vi "DOE Calculate Dryer EF.vi"(5 "Use Runtime RMC Calculation?":bool=TRUE, 7 "Dryer Initial IMC Data in":T7 {"Maximum Weight (lbf)" format="%03_6g"; "Average Weight (lbf)" format="%03_6g"; "Minimum Weight (lbf)" format="%03_6g"; "CEF (lbf/kWh)" format="%03_6g"; "Actual Final RMC (%)" format="%03_6g"; "Tolerance(%)" format="%0#_6g"; "Bone Dry Wt(lbs)" format="%03_6g"; "RMC (Desired %)" format="%0#_6g"; "Actual Initial RMC (%)" format="%03_6g"; "Measured IMC (lbs)" format="%0#_6g"}, 8 "Error In":errorcluster, 11 "Measurments":T1 {"Power Measurements"."Voltage (V):Element 1 Avg" format="%.3g"; "Power Measurements"."Voltage (V):Element 2 Avg" format="%.3g"; "Power Measurements"."Max Watt Hours" format="%.3g"; "Power Measurements"."Power Factor:Element 2" format="%.3g"; "Power Measurements"."Power Factor:Element 1" format="%.3g"; "Power Measurements"."Apparent Power (VA):Element 2" format="%.3g"; "Power Measurements"."Apparent Power (VA):Element 1" format="%.3g"; "Power Measurements"."Frequency (Hz):Element 1" format="%.3g"; "Power Measurements"."Time:Element 1" format="%.3g"; "Power Measurements"."Voltage Crest Factor:Element 2" format="%.3g"; "Power Measurements"."Voltage Crest Factor:Element 1" format="%.3g"; "Power Measurements"."Voltage Harmonic (%):Element 2" format="%.3g"; "Power Measurements"."Voltage Harmonic (%):Element 1" format="%.3g"; "Power Measurements"."Current Crest Factor:Element 2" format="%.3g"; "Power Measurements"."Current Crest Factor:Element 1" format="%.3g"; "Power Measurements"."Voltage (V):Element 1" format="%.3g"; "Power Measurements"."Voltage (V):Element 2" format="%.3g"; "Power Measurements"."Watt Hours (Wh):Sigma" format="%.3f"; "Power Measurements"."Power (W):Sigma" format="%.3g"; "Power Measurements"."Current (A):Element 2" format="%.3e"; "Power Measurements"."Current (A):Element 1" format="%.3e"}) -> (0 "Error Out":errorcluster, 1 "RMC Data":string[][](array[string]), 2 "Dryer Initial IMC Data out":T7 {"Maximum Weight (lbf)" format="%03_6g"; "Average Weight (lbf)" format="%03_6g"; "Minimum Weight (lbf)" format="%03_6g"; "CEF (lbf/kWh)" format="%03_6g"; "Actual Final RMC (%)" format="%03_6g"; "Tolerance(%)" format="%0#_6g"; "Bone Dry Wt(lbs)" format="%03_6g"; "RMC (Desired %)" format="%0#_6g"; "Actual Initial RMC (%)" format="%03_6g"; "Measured IMC (lbs)" format="%0#_6g"}, 3 "Measurments Out":T1 {"Power Measurements"."Voltage (V):Element 1 Avg" format="%.3g"; "Power Measurements"."Voltage (V):Element 2 Avg" format="%.3g"; "Power Measurements"."Max Watt Hours" format="%.3g"; "Power Measurements"."Power Factor:Element 2" format="%.3g"; "Power Measurements"."Power Factor:Element 1" format="%.3g"; "Power Measurements"."Apparent Power (VA):Element 2" format="%.3g"; "Power Measurements"."Apparent Power (VA):Element 1" format="%.3g"; "Power Measurements"."Frequency (Hz):Element 1" format="%.3g"; "Power Measurements"."Time:Element 1" format="%.3g"; "Power Measurements"."Voltage Crest Factor:Element 2" format="%.3g"; "Power Measurements"."Voltage Crest Factor:Element 1" format="%.3g"; "Power Measurements"."Voltage Harmonic (%):Element 2" format="%.3g"; "Power Measurements"."Voltage Harmonic (%):Element 1" format="%.3g"; "Power Measurements"."Current Crest Factor:Element 2" format="%.3g"; "Power Measurements"."Current Crest Factor:Element 1" format="%.3g"; "Power Measurements"."Voltage (V):Element 1" format="%.3g"; "Power Measurements"."Voltage (V):Element 2" format="%.3g"; "Power Measurements"."Watt Hours (Wh):Sigma" format="%.3f"; "Power Measurements"."Power (W):Sigma" format="%.3g"; "Power Measurements"."Current (A):Element 2" format="%.3e"; "Power Measurements"."Current (A):Element 1" format="%.3e"})   [LabVIEW 2020]
uses:
  Type Definitions/DOE Front Panel Meters.ctl
  Utility/Type Definitions/UTILITY Power Data.ctl
  Utility/Standby Power/Type Definitions/Standby Power Main Data.ctl
  Drivers/Omega FMA-1600A Series Gas Flow Meter/Type Definitions/FMA1600A Gas Data.ctl
  Drivers/Omega FMA-1600A Series Gas Flow Meter/Type Definitions/FMA1600A Gas Type.ctl
  Range/Type Definitions/RANGE Meter Selector 1-2.ctl
  Utility/Save File/File Setup (Public)/Type Definition/DPT IMC Data.ctl
  Type Definitions/DOE Dryer Standard.ctl
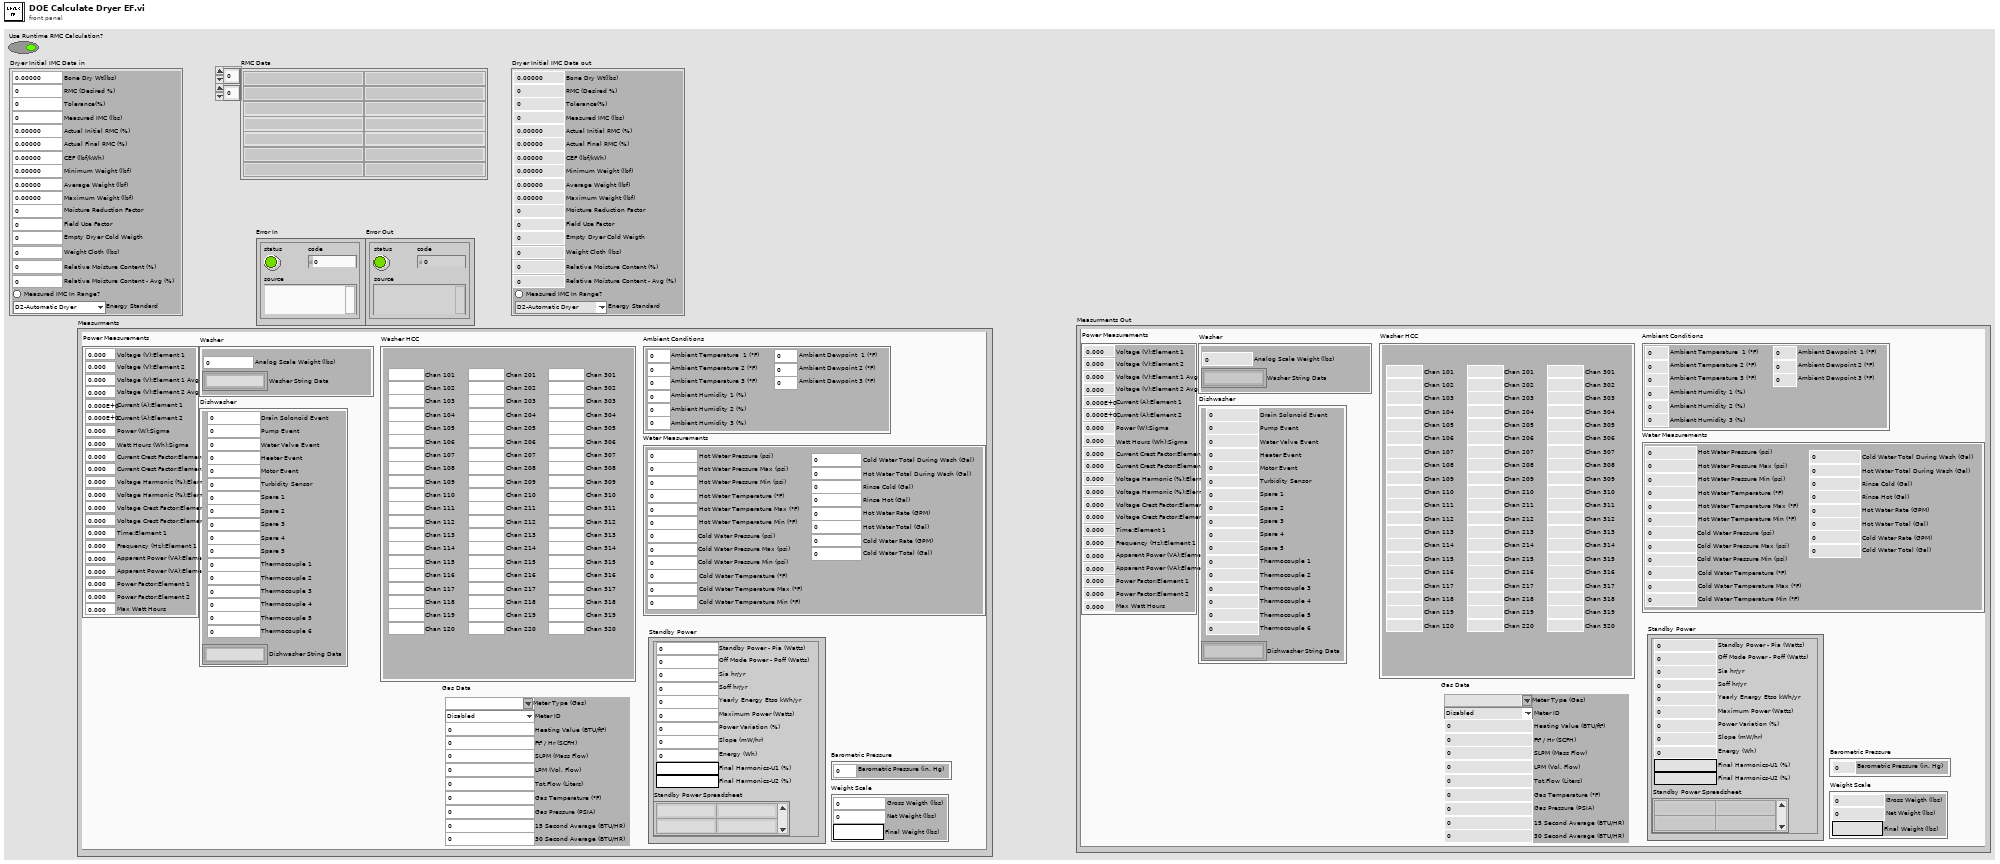
[diagram p1: front panel]
types:
  T1 = typedef "DOE Front Panel Meters.ctl" = cluster{"Power Measurements":T2, "Standby Power":T3, "Washer":cluster{"Washer String Data":string[][], "Analog Scale Weight (lbs)":dbl}, "Dishwasher":cluster{"Drain Solonoid Event":i32, "Pump Event":i32, "Water Valve Event":i32, "Heater Event":i32, "Motor Event":i32, "Turbidity Sensor":dbl, "Spare 2":dbl, "Spare 3":dbl, "Spare 4":dbl, "Spare 5":dbl, "Thermocouple 1":dbl, "Thermocouple 2":dbl, "Thermocouple 3":dbl, "Thermocouple 4":dbl, "Thermocouple 5":dbl, "Thermocouple 6":dbl, "Spare 1":dbl, "Dishwasher String Data":string[][]}, "Washer HCC":cluster{"Chan 101":dbl, "Chan 102":dbl, "Chan 103":dbl, "Chan 104":dbl, "Chan 105":dbl, "Chan 106":dbl, "Chan 107":dbl, "Chan 108":dbl, "Chan 109":dbl, "Chan 110":dbl, "Chan 111":dbl, "Chan 112":dbl, "Chan 113":dbl, "Chan 114":dbl, "Chan 115":dbl, "Chan 116":dbl, "Chan 117":dbl, "Chan 118":dbl, "Chan 119":dbl, "Chan 120":dbl, "Chan 201":dbl, "Chan 202":dbl, "Chan 203":dbl, "Chan 204":dbl, "Chan 205":dbl, "Chan 206":dbl, "Chan 207":dbl, "Chan 208":dbl, "Chan 209":dbl, "Chan 210":dbl, "Chan 211":dbl, "Chan 212":dbl, "Chan 213":dbl, "Chan 214":dbl, "Chan 215":dbl, "Chan 216":dbl, "Chan 217":dbl, "Chan 218":dbl, "Chan 219":dbl, "Chan 220":dbl, "Chan 301":dbl, "Chan 302":dbl, "Chan 303":dbl, "Chan 304":dbl, "Chan 305":dbl, "Chan 306":dbl, "Chan 307":dbl, "Chan 308":dbl, "Chan 309":dbl, "Chan 310":dbl, "Chan 311":dbl, "Chan 312":dbl, "Chan 313":dbl, "Chan 314":dbl, "Chan 315":dbl, "Chan 316":dbl, "Chan 317":dbl, "Chan 318":dbl, "Chan 319":dbl, "Chan 320":dbl}, "Barometric Pressure":cluster{"Barometric Pressure (in. Hg)":dbl}, "Ambient Conditions":cluster{"Ambient Temperature  1 (°F)":dbl, "Ambient Temperature 2 (°F)":dbl, "Ambient Temperature 3 (°F)":dbl, "Ambient Humidity 1 (%)":dbl, "Ambient Humidity 2 (%)":dbl, "Ambient Humidity 3 (%)":dbl, "Ambient Dewpoint  1 (°F)":dbl, "Ambient Dewpoint 2 (°F)":dbl, "Ambient Dewpoint 3 (°F)":dbl}, "Weight Scale":cluster{"Gross Weigth (lbs)":dbl, "Net Weight (lbs)":dbl, "Final Weight (lbs)":string}, "Water Measurements":cluster{"Hot Water Pressure (psi)":dbl, "Hot Water Pressure Max (psi)":dbl, "Hot Water Temperature (°F)":dbl, "Cold Water Pressure (psi)":dbl, "Cold Water Pressure Max (psi)":dbl, "Hot Water Temperature Max (°F)":dbl, "Cold Water Temperature (°F)":dbl, "Cold Water Temperature Max (°F)":dbl, "Hot Water Total (Gal)":dbl, "Hot Water Rate (GPM)":dbl, "Cold Water Total (Gal)":dbl, "Cold Water Rate (GPM)":dbl, "Cold Water Total During Wash (Gal)":dbl, "Hot Water Total During Wash (Gal)":dbl, "Rinse Cold (Gal)":dbl, "Rinse Hot (Gal)":dbl, "Hot Water Pressure Min (psi)":dbl, "Hot Water Temperature Min (°F)":dbl, "Cold Water Pressure Min (psi)":dbl, "Cold Water Temperature Min (°F)":dbl}, "Gas Data":T4}
  T2 = typedef "UTILITY Power Data.ctl" = cluster{"Current (A):Element 1":dbl, "Current (A):Element 2":dbl, "Power (W):Sigma":dbl, "Watt Hours (Wh):Sigma":dbl, "Voltage (V):Element 2":dbl, "Voltage (V):Element 1":dbl, "Current Crest Factor:Element 1":dbl, "Current Crest Factor:Element 2":dbl, "Voltage Harmonic (%):Element 1":dbl, "Voltage Harmonic (%):Element 2":dbl, "Voltage Crest Factor:Element 1":dbl, "Voltage Crest Factor:Element 2":dbl, "Time:Element 1":dbl, "Frequency (Hz):Element 1":dbl, "Apparent Power (VA):Element 1":dbl, "Apparent Power (VA):Element 2":dbl, "Power Factor:Element 1":dbl, "Power Factor:Element 2":dbl, "Max Watt Hours":dbl, "Voltage (V):Element 2 Avg":dbl, "Voltage (V):Element 1 Avg":dbl}
  T3 = typedef "Standby Power Main Data.ctl" = cluster{"Standby Power Spreadsheet":string[][], "Standby Power - Pia (Watts)":dbl, "Off Mode Power - Poff (Watts)":dbl, "Sia hr/yr":dbl, "Soff hr/yr":dbl, "Yearly Energy Etso kWh/yr":dbl, "Maximum Power (Watts)":dbl, "Power Variation (%)":dbl, "Slope (mW/hr)":dbl, "Final Harmonics-U1 (%)":string, "Final Harmonics-U2 (%)":string, "Energy (Wh)":dbl}
  T4 = typedef "FMA1600A Gas Data.ctl" = cluster{"Meter Type (Gas)":T5, "Meter ID":T6, "Heating Value (BTU/ft³)":dbl, "Ft³ / Hr (SCFH)":dbl, "15 Second Average (BTU/HR)":dbl, "30 Second Average (BTU/HR)":dbl, "SLPM (Mass Flow)":dbl, "LPM (Vol. Flow)":dbl, "Gas Temperature (°F)":dbl, "Gas Pressure (PSIA)":dbl, "Tot.Flow (Liters)":dbl}
  T5 = typedef "FMA1600A Gas Type.ctl" = string
  T6 = typedef "RANGE Meter Selector 1-2.ctl" = enum16{"Disabled", "Meter 1", "Meter 2", "Auto"}
  T7 = typedef "DPT IMC Data.ctl" = cluster{"Measured IMC (lbs)":dbl, "Actual Initial RMC (%)":dbl, "RMC (Desired %)":dbl, "Bone Dry Wt(lbs)":dbl, "Tolerance(%)":dbl, "Actual Final RMC (%)":dbl, "CEF (lbf/kWh)":dbl, "Minimum Weight (lbf)":dbl, "Average Weight (lbf)":dbl, "Maximum Weight (lbf)":dbl, "Measured IMC In Range?":bool, "Moisture Reduction Factor":dbl, "Field Use Factor":dbl, "Empty Dryer Cold Weigth":dbl, "Energy Standard":T8, "Weight Cloth (lbs)":dbl, "Relative Moisture Content (%)":dbl, "Relative Moisture Content - Avg (%)":dbl}
  T8 = typedef "DOE Dryer Standard.ctl" = enum16{"D2-Automatic Dryer", "D2-Timer Dryer", "D1-Automatic Dryer", "D1-Timer Dryer", "Other"}
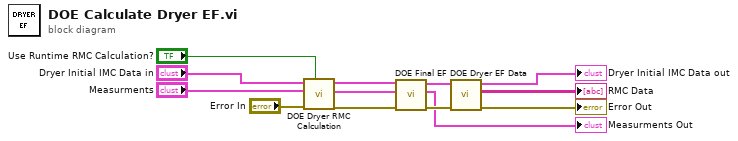
[diagram p0: block diagram]
diagram:
  n1 = call "DOE Dryer RMC Calculation.vi"("Use Runtime RMC Calculation?"="Use Runtime RMC Calculation?", "Error In"="Error In", "Measurments"="Measurments", "Dryer Initial IMC Data Input"="Dryer Initial IMC Data in") -> ("Error Out"=w9:errorcluster, "Measurments Out"=w3:T1, "Dryer Initial IMC Data Output"=w11:T7)  [unwired: 5 in]
  n2 = call "DOE Final EF.vi"("Error In"=w9, "Measurments"=w3, "Dryer Initial IMC Data Input"=w11) -> ("Error Out"=w8:errorcluster, "Measurments Out"=→"Measurments Out":T1, "Dryer Initial IMC Data Output"=w7:T7)  [unwired: 6 in]
  n3 = call "DOE Dryer EF Data.vi"("Error In"=w8, "Dryer Initial IMC Data In"=w7) -> ("Error Out"=→"Error Out":errorcluster, "RMC Data"=→"RMC Data":string[][], "Dryer Initial IMC Data out"=→"Dryer Initial IMC Data out":T7)  [unwired: 7 in]
